vi "ForceSensComm.vi"() -> (0 "Daq Array":refnum<k21>[](array[refnum]), 1 "error out":errorcluster, 2 "Array1":sgl[][][](array[numeric]), 3 "Array":dbl[][](array[numeric]))   [LabVIEW 2011]
uses:
  <vilib>/DAQmx/read.llb/DAQmx Read (Analog 2D DBL NChan NSamp).vi
  <vilib>/DAQmx/create/channels.llb/DAQmx Create Channel (AI-Voltage-Basic).vi
  <vilib>/DAQmx/configure/timing.llb/DAQmx Timing (Sample Clock).vi
  <vilib>/DAQmx/configure/trigger.llb/DAQmx Start Trigger (Digital Edge).vi
  <vilib>/DAQmx/miscellaneous.llb/DAQmx Fill In Error Info.vi
panel:
  in  "Calibration FilesT1I1T2I2":path[](array[path])=[path "Z:/K1/Labview code Backup/FT11332.cal", path "Z:/K1/Labview code Backup/FT14967.cal", path "Z:/K1/Labview code Backup/FT5076.cal", path "Z:/K1/Labview code Backup/FT6214.cal"]
  in  "DAQ Devices":tag[](array[tag])=["Dev3", "Dev1", "Dev2", "Dev5"]
  in  "Sample Rate":dbl=1000.0
  in  "Buffer Size":i32=5000
  in  "Connection Mode":i32(ring)=-1 items=["default"=-1, "RSE"=10083, "NRSE"=10078, "Differential"=10106, "Pseudodifferential"=12529]
  in  "Channels":string[](array[string])=["0:5", "0:5", "0:5", "0:5"]
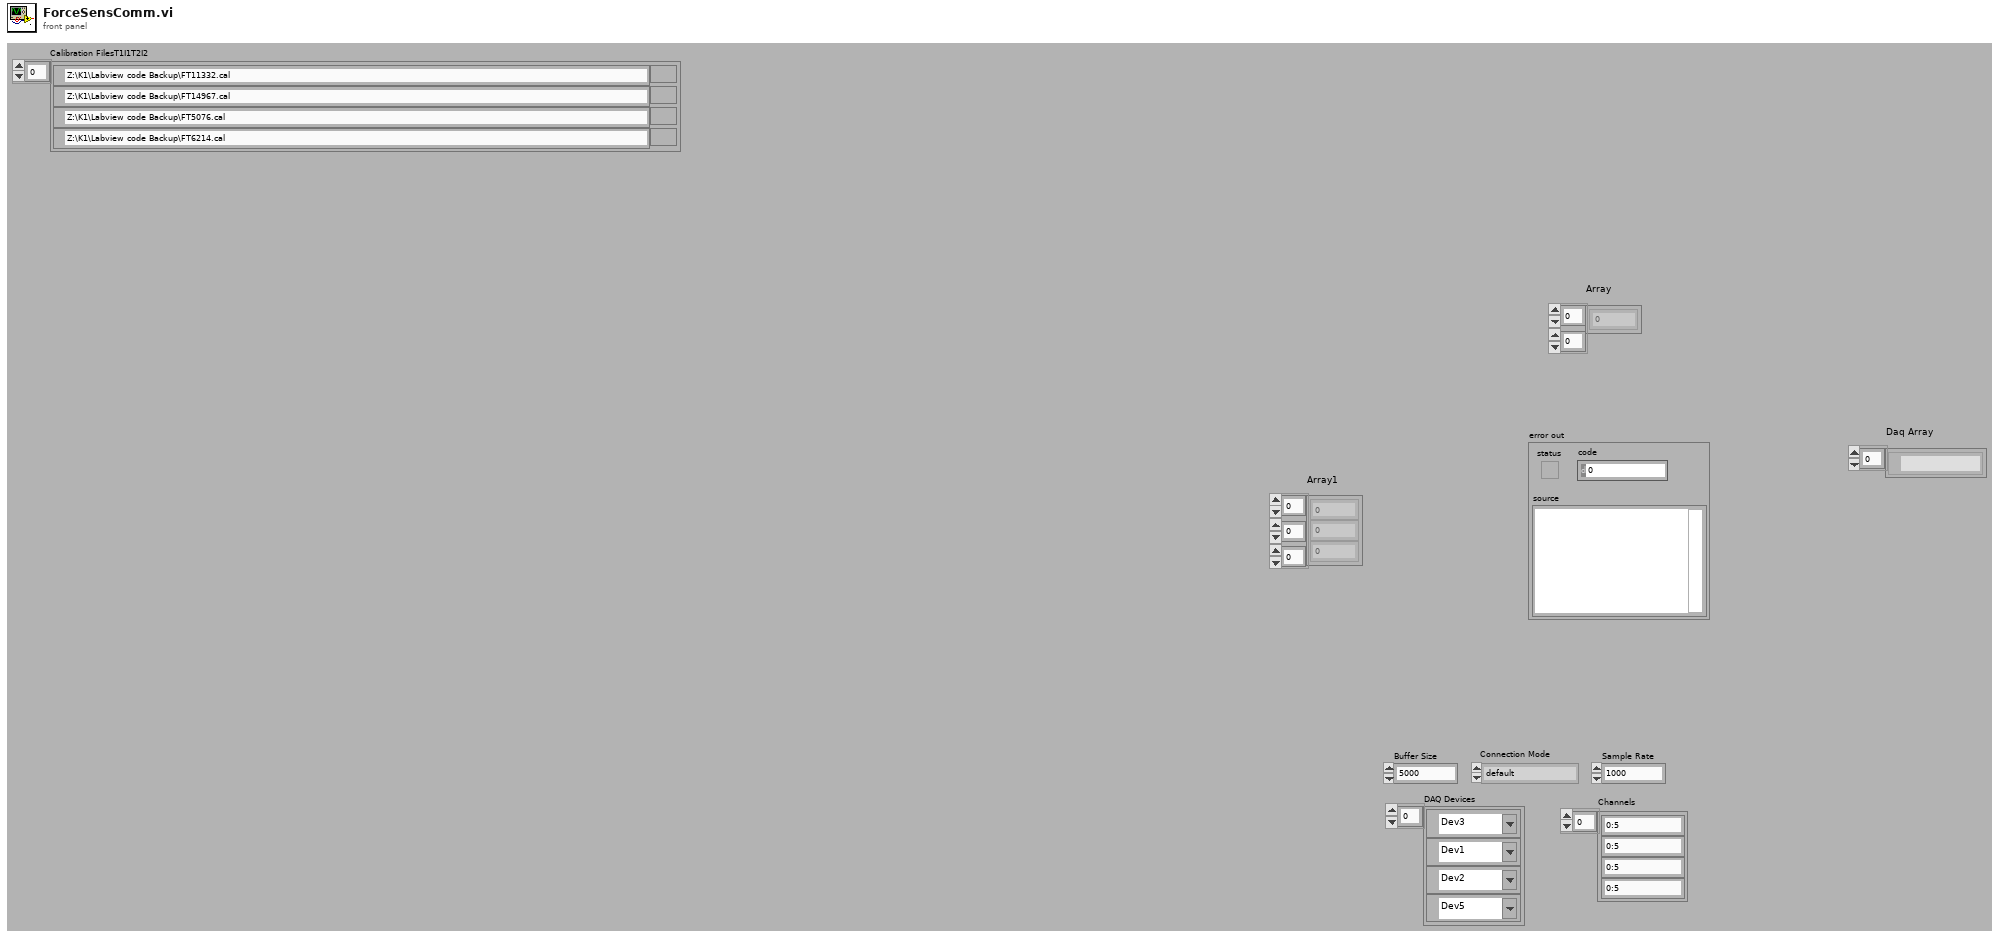
[diagram p1: front panel]
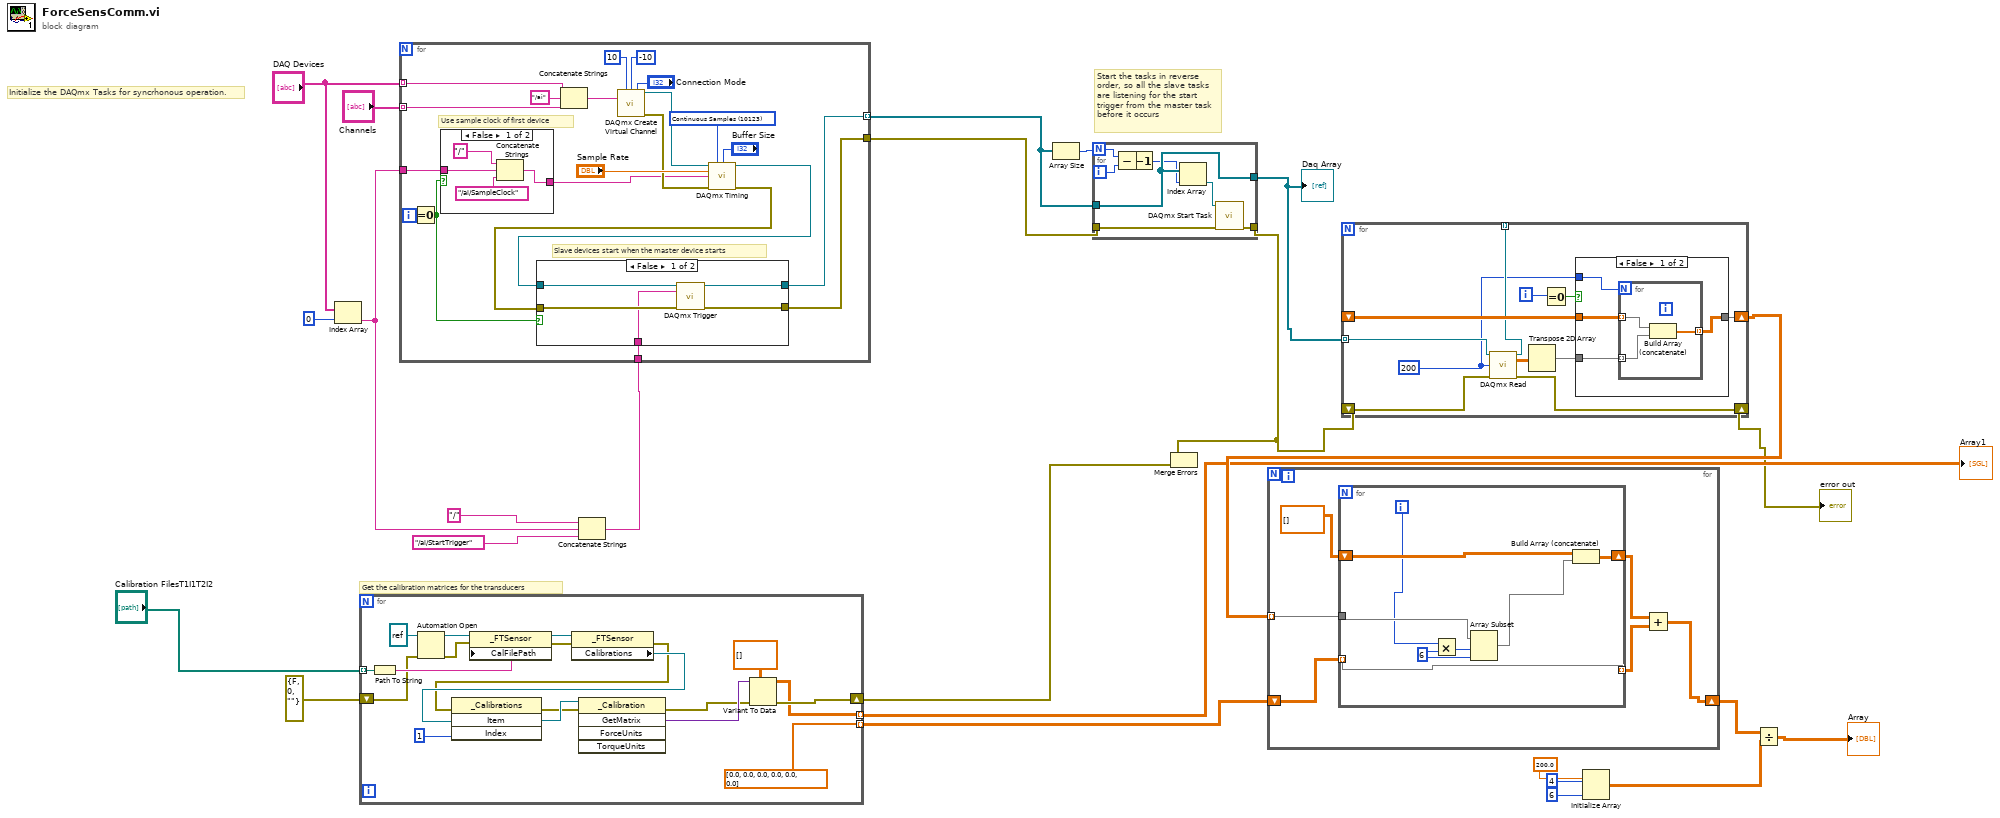
[diagram p0: block diagram]
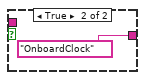
[diagram p3: hidden frame]
diagram:
  # "Initialize the DAQmx Tasks for syncrhonous operation."
  # "Get the calibration matrices for the transducers"
  # "Start the tasks in reverse order, so all the slave tasks are listening for the start trigger from the master task before it occurs"
  n1 = Index Array(array="DAQ Devices", index=0) -> (element=w22:tag)
  n2 = for {
    tunnel: "Calibration FilesT1I1T2I2" -> [w41] mode=indexing
    shift-right: [w32] -> w23
    shift-left: errorcluster {"status"=FALSE, "code"=0, "source"=""} ("error out") -> [w29]
    tunnel: [sgl[] [0.0, 0.0, 0.0, 0.0, 0.0, 0.0]] -> w12 mode=indexing
    tunnel: [w27] -> w4 mode=indexing
    n3 = Path To String(path=w41) -> (string=w40:string)
    n4 = Automation Open(error in (no error)=w29, Automation Refnum=refnum<k7> refnum ("ATIDAQFT._FTSensor")) -> (Automation Refnum=w30:refnum<k7>, error out=w26:errorcluster)  [unwired: 1 in, 1 out]
    n5 = property class="_FTSensor"(reference=w30, error in=w26, "CalFilePath"=w40) -> (reference out=w42:refnum<k7>, error out=w36:errorcluster)
    n6 = property class="_FTSensor"(reference=w42, error in=w36) -> (error out=w35:errorcluster, "Calibrations"=w44:refnum<k7>)  [unwired: 1 out]
    n7 = invoke class="_Calibrations" method="Item"(reference=w44, error in=w35, "Index"=1) -> (error out=w34:errorcluster, "Item"=w39:refnum<k7>)  [unwired: 1 in, 2 out]
    n8 = invoke class="_Calibration" method="GetMatrix"(reference=w39, error in=w34) -> (error out=w33:errorcluster, "GetMatrix"=w38:variant)  [unwired: 3 in, 3 out]
    n9 = Variant To Data(error in=w33, type=sgl[][] [], Variant=w38) -> (data=w27:sgl[][], error out=w32:errorcluster)
  }
  "Array1" <- w4
  n10 = Concatenate Strings("/", w22, "/ai/StartTrigger") -> (w19:string)
  n11 = for {
    tunnel: "DAQ Devices" -> [w65] mode=indexing
    tunnel: "Channels" -> [w64] mode=indexing
    tunnel: w19 -> [w55]
    tunnel: [w52] -> w20
    tunnel: w22 -> [w49]
    tunnel: [w45] -> w6 mode=indexing
    i -> [w57]
    w59 = 10123 items=["Finite Samples"=10178, "Continuous Samples"=10123, "Hardware Timed Single Point"=12522] ("sample mode")
    # "Slave devices start when the master device starts"
    # "Use sample clock of first device"
    n12 = Equal To 0?(x=w57) -> (x = 0?=w51:bool)
    n13 = case shown="False" w51 {
      tunnel: [w66 tag "OnboardClock"] -> w50
      tunnel: w49 -> [w67 _]
      frame False {
        n14 = Concatenate Strings("/", w67, "/ai/SampleClock") -> (w66:string)
      }
      frame True {
      }
    }
    n15 = Concatenate Strings(w65, "/ai", w64) -> (w62:string)
    n16 = call-poly <vilib>:"DAQmx Create Virtual Channel.vi"("maximum value"=10, "minimum value"=-10, "input terminal configuration"="Connection Mode", "physical channels"=w62) -> ("task out"=w61:refnum<k21>, "error out"=w54:errorcluster)  [unwired: 5 in, 5 out]
    n17 = call-poly <vilib>:"DAQmx Timing.vi"("task/channels in"=w61, "sample mode"=w59, "samples per channel"="Buffer Size", "rate"="Sample Rate", "source"=w50, "error in"=w54) -> ("task out"=w56:refnum<k21>, "error out"=w53:errorcluster)  [unwired: 1 in, 7 out]
    n18 = case shown="False" w51 {
      tunnel: w56 -> [w75 w77]
      tunnel: [w74 w77] -> w45
      tunnel: w55 -> [w71 _]
      tunnel: w53 -> [w73 w76]
      tunnel: [w72 w76] -> w52
      frame False {
        n19 = call-poly <vilib>:"DAQmx Trigger.vi"("task/channels in"=w75, "source"=w71, "error in"=w73) -> ("task out"=w74:refnum<k21>, "error out"=w72:errorcluster)  [unwired: 1 in, 10 out]
      }
      frame True {
      }
    }
  }
  n20 = Array Size(array=w6) -> (size(s)=w24:i32)
  n21 = for {
    N: w24 -> [w85]
    tunnel: w6 -> [w80]
    tunnel: w20 -> [w81]
    tunnel: [w80] -> w1
    tunnel: [w78] -> w14
    i -> [w84]
    n22 = Subtract(x=w85, y=w84) -> (x-y=w83:i32)
    n23 = Decrement(x=w83) -> (x-1=w79:i32)
    n24 = Index Array(array=w80, index=w79) -> (element=w82:refnum<k21>)
    n25 = call <vilib>:"DAQmx Start Task.vi"("task/channels in"=w82, "error in"=w81) -> ("error out"=w78:errorcluster)  [unwired: 13 out]
  }
  "Daq Array" <- w1
  n26 = Merge Errors(w14, w23) -> ()  [unwired: 1 out]
  n27 = for {
    tunnel: w1 -> [w96] mode=indexing
    shift-right: [w93] -> w2
    shift-left: w14 -> [w95]
    shift-right: [w90] -> w13
    shift-left: _ -> [w88]
    tunnel: [w87] -> _ mode=indexing
    i -> [w92]
    w86 = 200
    n28 = call-poly <vilib>:"DAQmx Read.vi"("task/channels in"=w96, "number of samples per channel"=w86, "error in"=w95) -> ("task out"=w87:refnum<k21>, "data"=w94:dbl[][], "error out"=w93:errorcluster)  [unwired: 10 out]
    n29 = Transpose 2D Array(2D array=w94) -> (transposed array=w89:dbl[][])
    n30 = Equal To 0?(x=w92) -> (x = 0?=w91:bool)
    n31 = case shown="False" w91 {
      tunnel: [w98 w104] -> w90
      tunnel: w89 -> [w99 w104]
      tunnel: w88 -> [w100 _]
      tunnel: w86 -> [w97 _]
      frame False {
        n32 = for {
          N: w97 -> [_]
          tunnel: w100 -> [w103] mode=indexing
          tunnel: w99 -> [w102] mode=indexing
          tunnel: [w101] -> w98 mode=indexing
          n33 = Build Array (concatenate)(w103, w102) -> (w101:dbl[])
        }
      }
      frame True {
      }
    }
  }
  "error out" <- w2
  n34 = for {
    tunnel: w13 -> [w110] mode=indexing
    shift-right: [w107] -> w11
    shift-left: w12 -> [w106]
    n35 = for {
      tunnel: w110 -> [w115]
      shift-right: [w114] -> w108
      shift-left: sgl[][] [] -> [w116]
      tunnel: [w113] -> w105 mode=indexing
      tunnel: w106 -> [w113] mode=indexing
      i -> [w112]
      w117 = 6
      n36 = Multiply(x=w112, y=w117) -> (x*y=w118:i32)
      n37 = Array Subset(array=w115, index=w118, length=w117) -> (w111:dbl[])
      n38 = Build Array (concatenate)(w116, w111) -> (w114:dbl[][])
    }
    n39 = Add ("Add.vi")(x=w108, y=w105) -> (x+y=w107:dbl[][])
  }
  n40 = Initialize Array(200.0 ("element"), 4 ("dimension size"), 6 ("dimension size")) -> (w7:dbl[][])
  n41 = Divide(x=w11, y=w7) -> (x/y=→"Array":dbl[][])
